vi "Message type.vi"(11 "IErrorHandler in":refnum<class "IErrorHandler.lvclass">) -> (2 "Internal message type":T1, 3 "IErrorHandler out":refnum<class "IErrorHandler.lvclass">)   [LabVIEW 2020, in "wamplv.lvlib" / "IErrorHandler.lvclass"]
uses:
  IErrorHandler.lvclass
  TypeDefs/Internal message type.ctl
  wamplv.lvlib
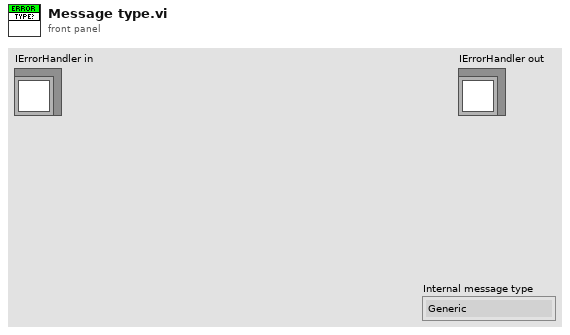
[diagram p1: front panel]
types:
  T1 = typedef "wamplv.lvlib/Internal message type.ctl" = enum16{"Generic", "Generic with write output", "Handle Result", "Handle Error", "Handle Abort"}
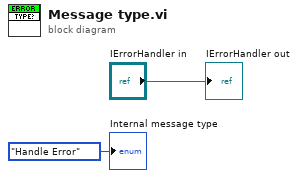
[diagram p0: block diagram]
diagram:
  "IErrorHandler out" <- "IErrorHandler in"
  "Internal message type" <- Internal_message_type."Handle Error" ("Internal message type")
